vi "convert_string_to_int64.vi"(3 "default (0)":i64, 4 "String in":string) -> (1 "int64 value out":i64)   [LabVIEW 2014, in "rszvl_rsidr_core.lvlib"]
uses:
  rszvl_rsidr_core.lvlib
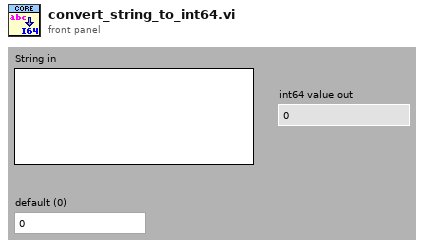
[diagram p1: front panel]
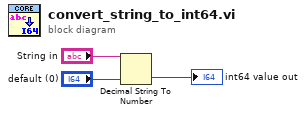
[diagram p0: block diagram]
diagram:
  n1 = Decimal String To Number(string="String in", default (0L)="default (0)") -> (number=→"int64 value out":i64)  [unwired: 1 in, 1 out]
